vi "Pre Launch Init.vi"(11 "Monitored Actor in":refnum<class "Monitored Actor.lvclass">) -> (0 "error out":errorcluster, 3 "Monitored Actor out":refnum<class "Monitored Actor.lvclass">)   [LabVIEW 2018, in "Monitored Actor.lvlib" / "Monitored Actor.lvclass"]
doc: "Sends a high priority message to it's self to notify the monitor that it's spawned. If it's in the runtime environment, this message is never sent, meaning the monitor will never spawn\n\nCopyright: MGI\nAuthored by: Derek Trepanier"
uses:
  Monitored Actor.lvclass
  C:/Program Files (x86)/National Instruments/LabVIEW 2018/vi.lib/ActorFramework/Actor/Actor.lvclass
  <vilib>/ActorFramework/Actor/Actor.lvclass/Actor.ctl
  <vilib>/ActorFramework/Message Enqueuer/Message Enqueuer.lvclass/Message Enqueuer.ctl
  <vilib>/ActorFramework/Message Enqueuer/Message Priority.ctl
  <vilib>/ActorFramework/Message Enqueuer/Enqueue.vi
  <vilib>/ActorFramework/Message Enqueuer/Init from Existing Queue.vi
  Monitored Actor Messages/Notify Monitor Msg/Notify Monitor Msg.lvclass
  C:/Program Files (x86)/National Instruments/LabVIEW 2018/vi.lib/ActorFramework/Message/Message.lvclass
  <vilib>/ActorFramework/Message Priority Queue/Priority Enqueue.vi
  <vilib>/ActorFramework/Actor/Actor.lvclass
  <vilib>/ActorFramework/Message Enqueuer/Message Enqueuer.lvclass
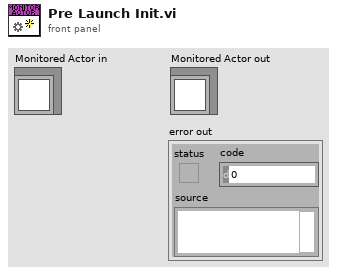
[diagram p1: front panel]
types:
  T1 = typedef "Actor Framework.lvlib/Message Enqueuer.lvclass/Message Priority.ctl" = enum16{"Low", "Normal", "High"}
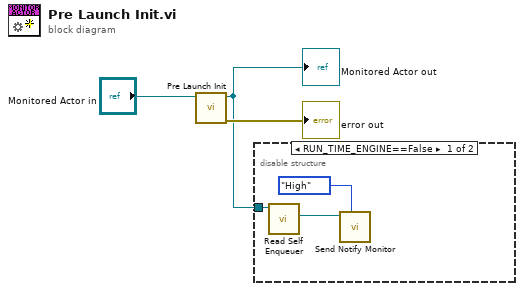
[diagram p0: block diagram]
diagram:
  n1 = call-parent "Pre Launch Init.vi"("Actor in"="Monitored Actor in") -> ("error out"=→"error out":errorcluster, "Actor out"=w1:refnum<class "Monitored Actor.lvclass">)  [unwired: 9 in]
  "Monitored Actor out" <- w1
  n2 = disable-structure shown="RUN_TIME_ENGINE==False" {
    disable-tunnel: w1 -> [w6 _]
    frame condition #0 (active) {
      n3 = call <vilib>:"Read Self Enqueuer.vi"("Actor"=w6) -> ("Self Enqueuer"=w5:refnum<class "Message Enqueuer.lvclass">)  [unwired: 10 in]
      n4 = call "Send Notify Monitor.vi"("Message Priority (Normal)"=Message_Priority."High", "Message Enqueuer"=w5) -> ()  [unwired: 8 in, 2 out]
    }
    frame condition #1 {
    }
  }
